vi "Seconds to phase offset.vi"(10 "Start of Laser":dbl, 11 "frequency":dbl) -> (3 "Phase":dbl)   [LabVIEW 2015]
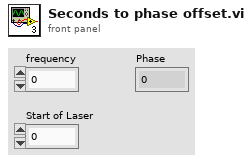
[diagram p1: front panel]
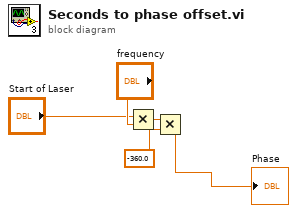
[diagram p0: block diagram]
diagram:
  n1 = Multiply(x="Start of Laser", y="frequency") -> (x*y=w3:dbl)
  n2 = Multiply(x=w3, y=-360.0) -> (x*y=→"Phase":dbl)
